vi "Prerun.vi"(8 "error in (no error)":errorcluster) -> (0 "error out":errorcluster)   [LabVIEW 2017, in "loggingModule.lvlib"]
doc: "This VI obtains the queue reference for the Logging module.\n\nQueue = messages from all modules to the Logging Module"
uses:
  loggingModule.lvlib
  Queue/TypeDefs/queueFGVState.ctl
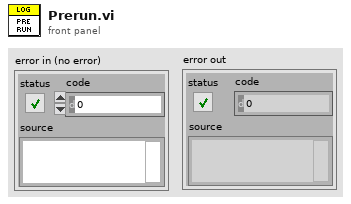
[diagram p1: front panel]
types:
  T1 = typedef "loggingModule.lvlib/queueFGVState.ctl" = enum16{"obtain", "enqueue low priority", "enqueue high priority", "dequeue", "release"}
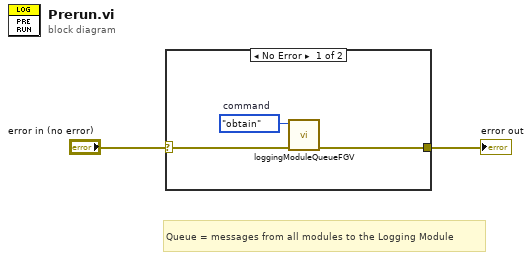
[diagram p0: block diagram]
diagram:
  # "Queue = messages from all modules to the Logging Module"
  n1 = case shown="No Error" "error in (no error)" {
    selector: "error in (no error)" -> [w5 w6]
    tunnel: [w4 w6] -> w1
    frame No Error {
      w3 = queueFGVState."obtain"  # command
      n2 = call "loggingModuleQueueFGV.vi"("error in (no error)"=w5, "command"=w3) -> ("error out"=w4:errorcluster)  [unwired: 8 in, 1 out]
    }
    frame Error {
    }
  }
  "error out" <- w1
